vi "Load Document.vi"(0 "Document In":refnum<class "Document.lvclass">, 1 "Path":path, 5 "error in (no error)":errorcluster) -> (14 "Document Out":refnum<class "Document.lvclass">, 15 "xml":string, 19 "error out":errorcluster)   [LabVIEW 2013, in "Document.lvclass"]
uses:
  Document.lvclass
  Document.lvclass/Document.ctl
  <userlib>/_OpenG.lib/lvzip/lvzip.llb/ZLIB Open Unzip Archive__ogtk.vi
  <userlib>/_OpenG.lib/lvzip/lvzip.llb/ZLIB Extract Stream__ogtk.vi
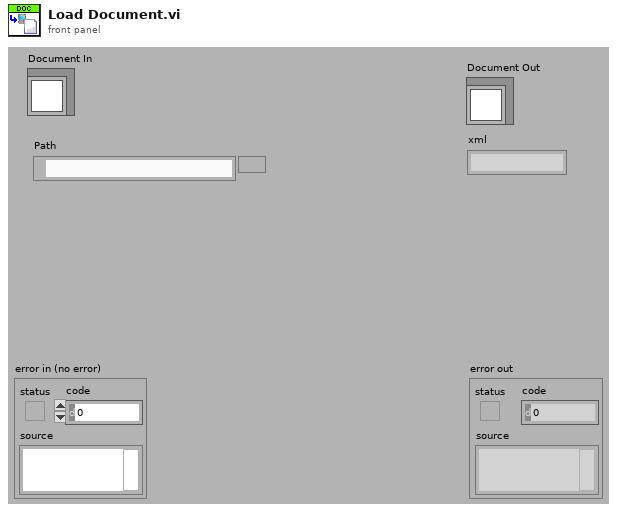
[diagram p1: front panel]
types:
  T1 = typedef "ZLIB Unzip Handle__ogtk.ctl" = refnum<k1>
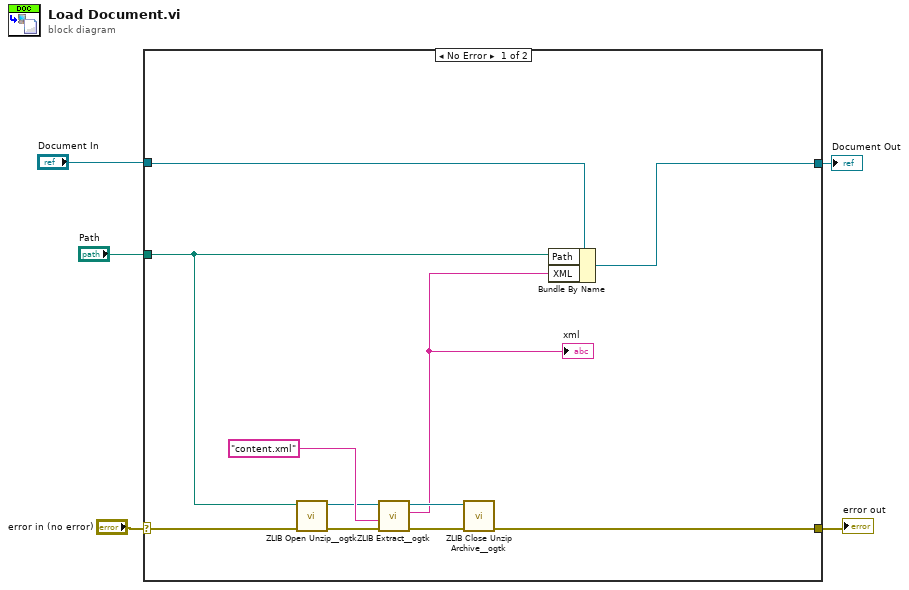
[diagram p0: block diagram]
diagram:
  n1 = case shown="No Error" "error in (no error)" {
    selector: "error in (no error)" -> [w11 w18]
    tunnel: [w7 w18] -> w4
    tunnel: [w15 w17] -> w1
    tunnel: "Document In" -> [w16 w17]
    tunnel: "Path" -> [w10 _]
    frame No Error {
      n2 = call-poly <userlib>:"ZLIB Open Unzip__ogtk.vi"("error in (no error)"=w11, "archive name"=w10) -> ("error out"=w12:errorcluster, "unzip Refnum"=w13:T1)  [unwired: 4 in]
      n3 = call-poly <userlib>:"ZLIB Extract__ogtk.vi"("error in (no error)"=w12, "internal name"="content.xml" ("name (empty: -)"), "unzip Refnum"=w13) -> ("error out"=w8:errorcluster, "byte stream"=w6:string, "unzip Refnum out"=w9:T1)  [unwired: 4 in]
      "xml" <- w6
      n4 = call <userlib>:"ZLIB Close Unzip Archive__ogtk.vi"("error in (no error)"=w8, "unzip Refnum"=w9) -> ("error out"=w7:errorcluster)  [unwired: 5 in]
      n5 = Bundle By Name(cluster=w16, "Path"=w10, "XML"=w6) -> (w15:refnum<class "Document.lvclass">)
    }
    frame Error {
    }
  }
  "error out" <- w4
  "Document Out" <- w1
